vi "FTW-Supervisor-Launch.vi"(5 "FTW Supervisor Configuration":string="{\n  \"AppName\":         \"Your Application\",\n  \"AppVersionMajor\": 0,\n  \"AppVersionMinor\": 0,\n  \"AppVersionPatch\": 1,\n  \"Identity\":        \"FTW Application Supervisor\",\n  \"InboxAddress\":    \"tcp://127.0.0.1:38900\",\n  \"DashboardInboxAddress\":     \"ws://127.0.0.1:38901\",\n  \"DashboardPublisherAddress\": \"ws://127.0.0.1:38902\",\n  \"DashboardPageAddress\":      \"ws://127.0.0.1:38903\",\n  \"LogRetentionPolicy\": {\n    \"PersistToDisk\": true,\n    \"LogFilepath\": \"%LocalAppData%/Featherweight/FTWApplicationLog.db\",\n    \"MaxEventsToKeep\": 100000,\n    \"MaxActorsToRemember\": 1000\n  }\n}", 11 "error in":errorcluster) -> (4 "FTW Supervisor Connection":refnum<class "FTW-Supervisor-Connector.lvclass">, 6 "Supervisor Address":string, 15 "error out":errorcluster)   [LabVIEW 2014, in "FTW-Supervisor.lvclass"]
uses:
  FTW-Supervisor.lvclass
  connector/FTW-Supervisor-Connector.lvclass
  connector/FTW-Actor-Connector.lvclass
panel:
  # "Inputs"
  # "Outputs"
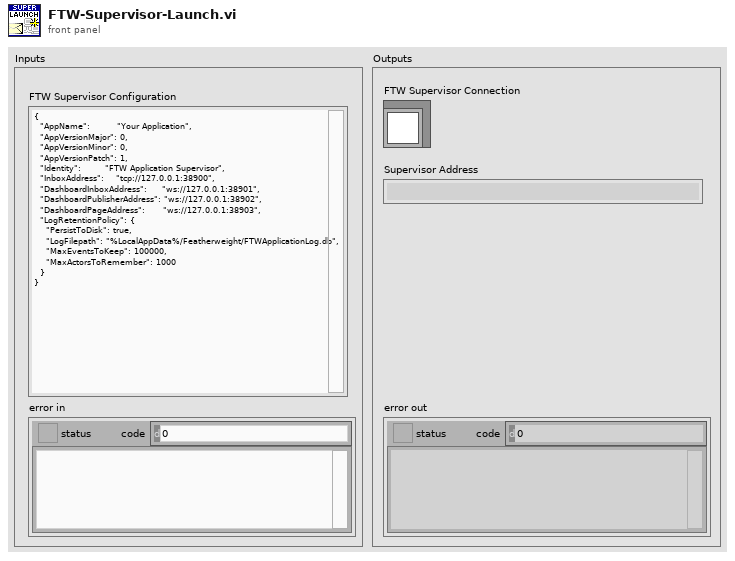
[diagram p1: front panel]
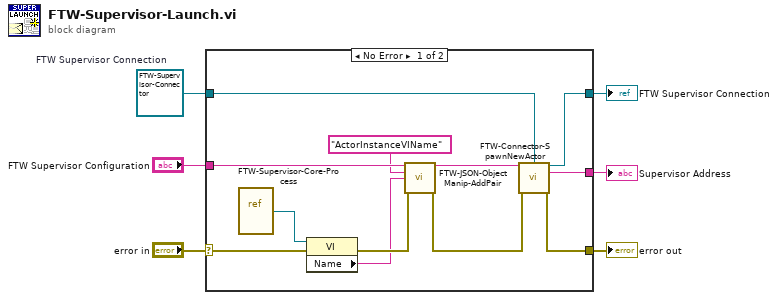
[diagram p0: block diagram]
diagram:
  w3 = refnum<class "FTW-Supervisor-Connector.lvclass"> refnum  # FTW Supervisor Connection
  n1 = case shown="No Error" "error in" {
    selector: "error in" -> [w15 w20]
    tunnel: [w17 w20] -> w6
    tunnel: [w18 w19] -> w4
    tunnel: w3 -> [w8 w19]
    tunnel: "FTW Supervisor Configuration" -> [w14 _]
    tunnel: [w7 _] -> w1
    frame No Error {
      n2 = vi-ref "FTW-Supervisor-Core-Process.vi"() -> (w16:refnum<vi>)
      n3 = property class="VI"(reference=w16, error in=w15) -> (error out=w13:errorcluster, "Name"=w10:string)  [unwired: 1 out]
      n4 = call "FTW-JSON-ObjectManip-AddPair.vi"("Input JSON Object"=w14, "Key"="ActorInstanceVIName", "Value"=w10, "error in"=w13) -> ("Output JSON Object"=w9:string, "error out"=w12:errorcluster)  [unwired: 10 in]
      n5 = call "FTW-Connector-SpawnNewActor.vi"("Instance Configuration"=w9, "FTW Actor Connector Type"=w8, "error in"=w12) -> ("FTW Actor Connector"=w18:refnum<class "FTW-Supervisor-Connector.lvclass">, "Instance Inbox Address"=w7:string, "error out"=w17:errorcluster)  [unwired: 9 in, 1 out]
    }
    frame Error {
    }
  }
  "error out" <- w6
  "FTW Supervisor Connection" <- w4
  "Supervisor Address" <- w1
